vi "J1939 System Definition API_Example_Get J1939 CD Settings.vi"() -> ()   [LabVIEW 2013]
uses:
  J1939 System Definition API.lvlibp/APIs/System Definition API/Types/Remove Item - Frame Cluster.ctl
  J1939 System Definition API.lvlibp/Shared/Types/XNET Settings.ctl
  NationalInstruments.VeriStand.SystemDefinitionAPI
  J1939 System Definition API.lvlibp/APIs/System Definition API/Types/Remove Frame Action.ctl
  J1939 System Definition API.lvlibp/APIs/System Definition API/SubVIs/Get XNET Properties.vi
  J1939 System Definition API.lvlibp/APIs/System Definition API/SubVIs/Get Frames.vi
  J1939 System Definition API.lvlibp
  J1939 System Definition API.lvlibp/APIs/System Definition API/J1939 System Definition API Support.lvlib
  J1939 System Definition API.lvlibp/Shared/J1939 Addon Shared.lvlib
panel:
  in  "Path":path=path "C:/Users/Public/Documents/National Instruments/NI VeriStand 2011/Projects/DynamicallyCreatedProject/DynamicallyCreatedProject.nivssdf"
  out "Device Settings":T3(array[cluster]) {"J1939 XNET Settings"."Termination" items=["Off", "On"]}
  out "error out":errorcluster
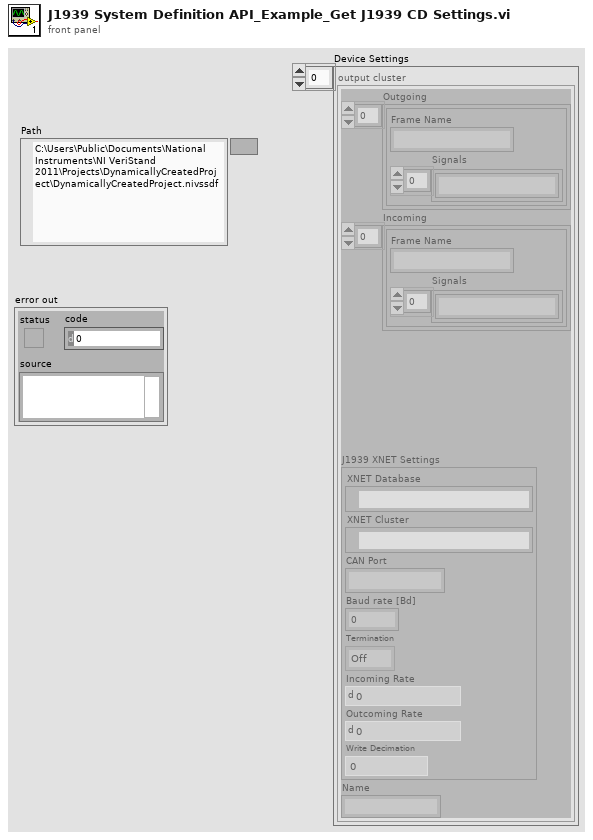
[diagram p1: front panel]
types:
  T1 = typedef "J1939 System Definition API.lvlibp/J1939 System Definition API Support.lvlib/Remove Item - Frame Cluster.ctl" = cluster{"Frame Name":string, "Signals":string[]}
  T2 = typedef "J1939 System Definition API.lvlibp/J1939 Addon Shared.lvlib/XNET Settings.ctl" = cluster{"XNET Database":refnum<k21>, "XNET Cluster":refnum<k21>, "CAN Port":string, "Baud rate [Bd]":u32, "Termination":u32, "Incoming Rate":u32, "Outcoming Rate":u32, "Write Decimation":u32}
  T3 = cluster{"Outgoing":T1[], "Incoming":T1[], "J1939 XNET Settings":T2, "Name":string}[]
  T4 = cluster{"Frame Array":T1[], "Frame Array":T1[], "J1939 XNET Settings":T2, "Name":string}[]
  T5 = typedef "J1939 System Definition API.lvlibp/J1939 System Definition API Support.lvlib/Remove Frame Action.ctl" = enum16{"Incoming", "Outgoing"}
  T6 = cluster{"Frame Array":T1[], "Frame Array":T1[], "J1939 XNET Settings":T2, "Name":string}
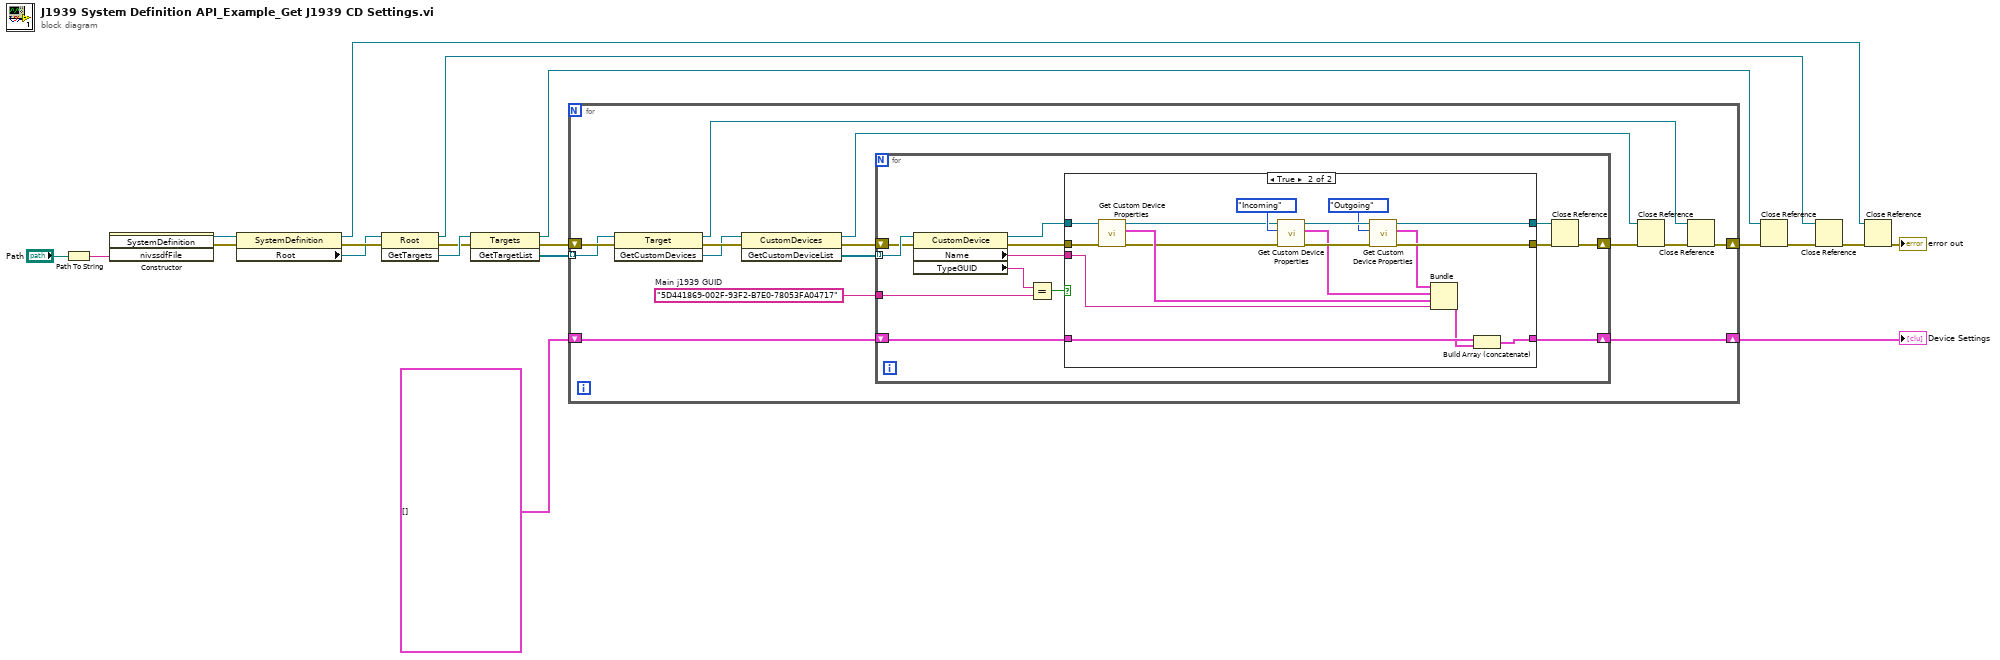
[diagram p0: block diagram]
diagram:
  n1 = Path To String(path="Path") -> (string=w13:string)
  n2 = constructor class="SystemDefinition"("nivssdfFile"=w13) -> (reference out=w16:refnum<k24>, error out=w18:errorcluster)  [unwired: 3 in, 2 out]
  n3 = property class="SystemDefinition"(reference=w16, error in=w18) -> (reference out=w5:refnum<k24>, error out=w17:errorcluster, "Root"=w14:refnum<k24>)
  n4 = invoke class="Root" method="GetTargets"(reference=w14, error in=w17) -> (reference out=w7:refnum<k24>, error out=w15:errorcluster, "GetTargets"=w19:refnum<k24>)  [unwired: 1 in]
  n5 = invoke class="Targets" method="GetTargetList"(reference=w19, error in=w15) -> (reference out=w9:refnum<k24>, error out=w12:errorcluster, "GetTargetList"=w10:refnum<k24>[])  [unwired: 1 in]
  n6 = for {
    tunnel: w10 -> [w21] mode=indexing
    shift-right: [w26] -> w11
    shift-left: w12 -> [w33]
    shift-right: [w23] -> w2
    shift-left: T4 [] ("Device Settings") -> [w22]
    w29 = "5D441869-002F-93F2-B7E0-78053FA04717"  # Main j1939 GUID
    n7 = invoke class="Target" method="GetCustomDevices"(reference=w21, error in=w33) -> (reference out=w20:refnum<k24>, error out=w32:errorcluster, "GetCustomDevices"=w31:refnum<k24>)  [unwired: 1 in]
    n8 = invoke class="CustomDevices" method="GetCustomDeviceList"(reference=w31, error in=w32) -> (reference out=w24:refnum<k24>, error out=w28:errorcluster, "GetCustomDeviceList"=w30:refnum<k24>[])  [unwired: 1 in]
    n9 = for {
      tunnel: w30 -> [w46] mode=indexing
      tunnel: w29 -> [w44]
      shift-right: [w38] -> w27
      shift-left: w28 -> [w42]
      shift-right: [w35] -> w23
      shift-left: w22 -> [w34]
      n10 = property class="CustomDevice"(reference=w46, error in=w42) -> (reference out=w45:refnum<k24>, error out=w41:errorcluster, "Name"=w36:string, "TypeGUID"=w37:string)
      n11 = Equal?(x=w37, y=w44) -> (x = y?=w43:bool)
      n12 = case shown="True" w43 {
        tunnel: w45 -> [w48 w63]
        tunnel: w41 -> [w49 w64]
        tunnel: [w49 w60] -> w40
        tunnel: [w48 w59] -> w39
        tunnel: w36 -> [_ w57]
        tunnel: [w47 w66] -> w35
        tunnel: w34 -> [w47 w65]
        frame False {
        }
        frame True {
          n13 = call-poly "Get Custom Device Properties.vi"("error in (no error)"=w64, "Custom Device ref in"=w63) -> ("error out"=w52:errorcluster, "J1939 XNET Settings"=w58:T2, "Custom Device ref out"=w51:refnum<k24>)  [unwired: 7 in]
          n14 = call-poly "Get Custom Device Properties.vi"("error in (no error)"=w52, "Action"=Remove_Frame_Action."Incoming", "Custom Device reference in"=w51) -> ("error out"=w61:errorcluster, "Frame Array"=w56:T1[], "Custom Device reference out"=w62:refnum<k24>)  [unwired: 6 in]
          n15 = call-poly "Get Custom Device Properties.vi"("error in (no error)"=w61, "Action"=Remove_Frame_Action."Outgoing", "Custom Device reference in"=w62) -> ("error out"=w60:errorcluster, "Frame Array"=w55:T1[], "Custom Device reference out"=w59:refnum<k24>)  [unwired: 6 in]
          n16 = Bundle("Frame Array"=w55, "Frame Array"=w56, "J1939 XNET Settings"=w58, "Name"=w57) -> (w50:T6)  [unwired: 1 in]
          n17 = Build Array (concatenate)(w65, w50) -> (w66:T4)
        }
      }
      n18 = Close Reference(reference=w39, error in (no error)=w40) -> (error out=w38:errorcluster)
    }
    n19 = Close Reference(reference=w24, error in (no error)=w27) -> (error out=w25:errorcluster)
    n20 = Close Reference(reference=w20, error in (no error)=w25) -> (error out=w26:errorcluster)
  }
  "Device Settings" <- w2
  n21 = Close Reference(reference=w9, error in (no error)=w11) -> (error out=w8:errorcluster)
  n22 = Close Reference(reference=w7, error in (no error)=w8) -> (error out=w6:errorcluster)
  n23 = Close Reference(reference=w5, error in (no error)=w6) -> (error out=→"error out":errorcluster)
